vi "add.vi"(8 "error in":errorcluster, 10 "label":string, 11 "labels in":refnum<class "labels.lvclass">) -> (0 "error out":errorcluster, 3 "labels out":refnum<class "labels.lvclass">)   [LabVIEW 2020, in "nominal types.lvlib" / "labels.lvclass"]
uses:
  labels.lvclass
  labels.lvclass/labels.ctl
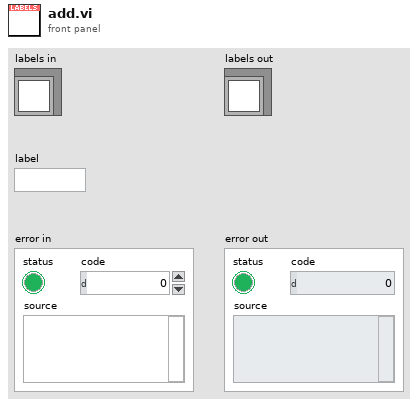
[diagram p1: front panel]
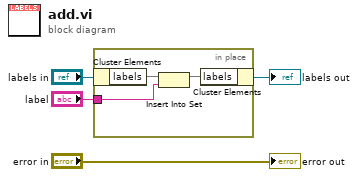
[diagram p0: block diagram]
diagram:
  n1 = in-place {
    in-place-border: "label" -> [w6]
    n2 = in-place-cluster #1("labels in") -> ("labels"=w7:set{string})
    n3 = Insert Into Set(10:w6, 11:w7) -> (3:w5:set{string})  [unwired: 1 out]
    n4 = in-place-cluster #1("labels"=w5) -> (→"labels out":refnum<class "labels.lvclass">)
  }
  "error out" <- "error in"
